vi "STM_Status.vi"() -> ()   [LabVIEW 2014]
uses:
  <userlib>/Nanonis Prog Interface V5/Nanonis Prog Interface.lvlib
panel:
  out "max value STM":dbl=1.6219152410013038e-10
  out "max value prep":dbl=2.1490820234504326e-10
  in  "Emission Current":u16(ring) items=["10", "1", "0.1"]
  out "STM [mBar]":dbl=1.554608664022794e-10 format="%#.2g"
  out "Prep [mBar]":dbl=2.1460036525589032e-10 format="%#.2g"
  out "Pressure":cluster{timestamp[], dbl[]}[](graph)=[{[timestamp(3559596166.680481 s since 1904-01-01), timestamp(3559596187.2546577 s since 1904-01-01)], [1.6219152410013038e-10, 1.5602781566759205e-10]}, {[timestamp(3559596166.680481 s since 1904-01-01), timestamp(3559596187.2546577 s since 1904-01-01)], [2.1490820234504326e-10, 2.1469723221478887e-10]}]
  in  "Resolution P":dbl=0.1
  in  "force update":dbl=20.0
  out "Cryo [K]":dbl=4.220807947684371 format="%#.2g"
  out "STM [K]":dbl=4.597361930995425 format="%#.2g"
  in  "Resolution Temp":dbl=0.1
  out "Temperature":cluster{timestamp[], dbl[]}[](graph)=[{[timestamp(3559596166.680481 s since 1904-01-01), timestamp(3559596187.2546577 s since 1904-01-01)], [4.221571920530717, 4.221402148787085]}, {[timestamp(3559596166.680481 s since 1904-01-01), timestamp(3559596187.2546577 s since 1904-01-01)], [4.572162263240161, 4.589400389803902]}]
  in  "Clear chart":bool
  in  "stop":bool
  in  "refresh":dbl=1.0
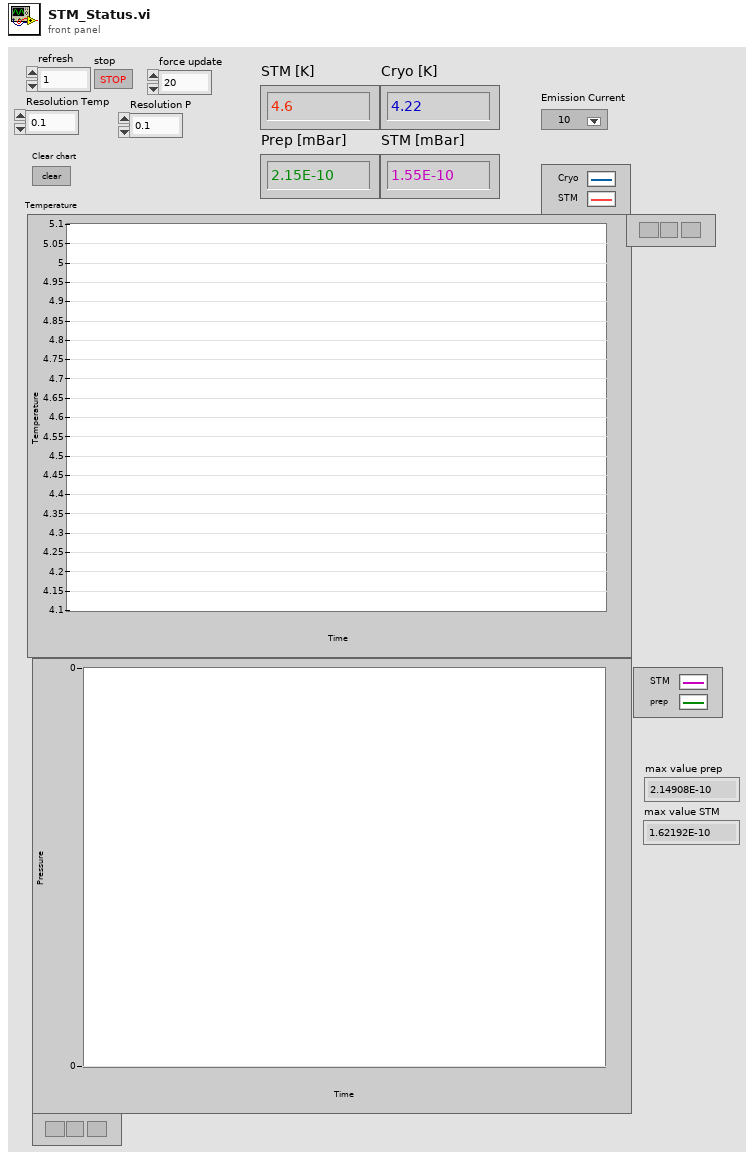
[diagram p1: front panel]
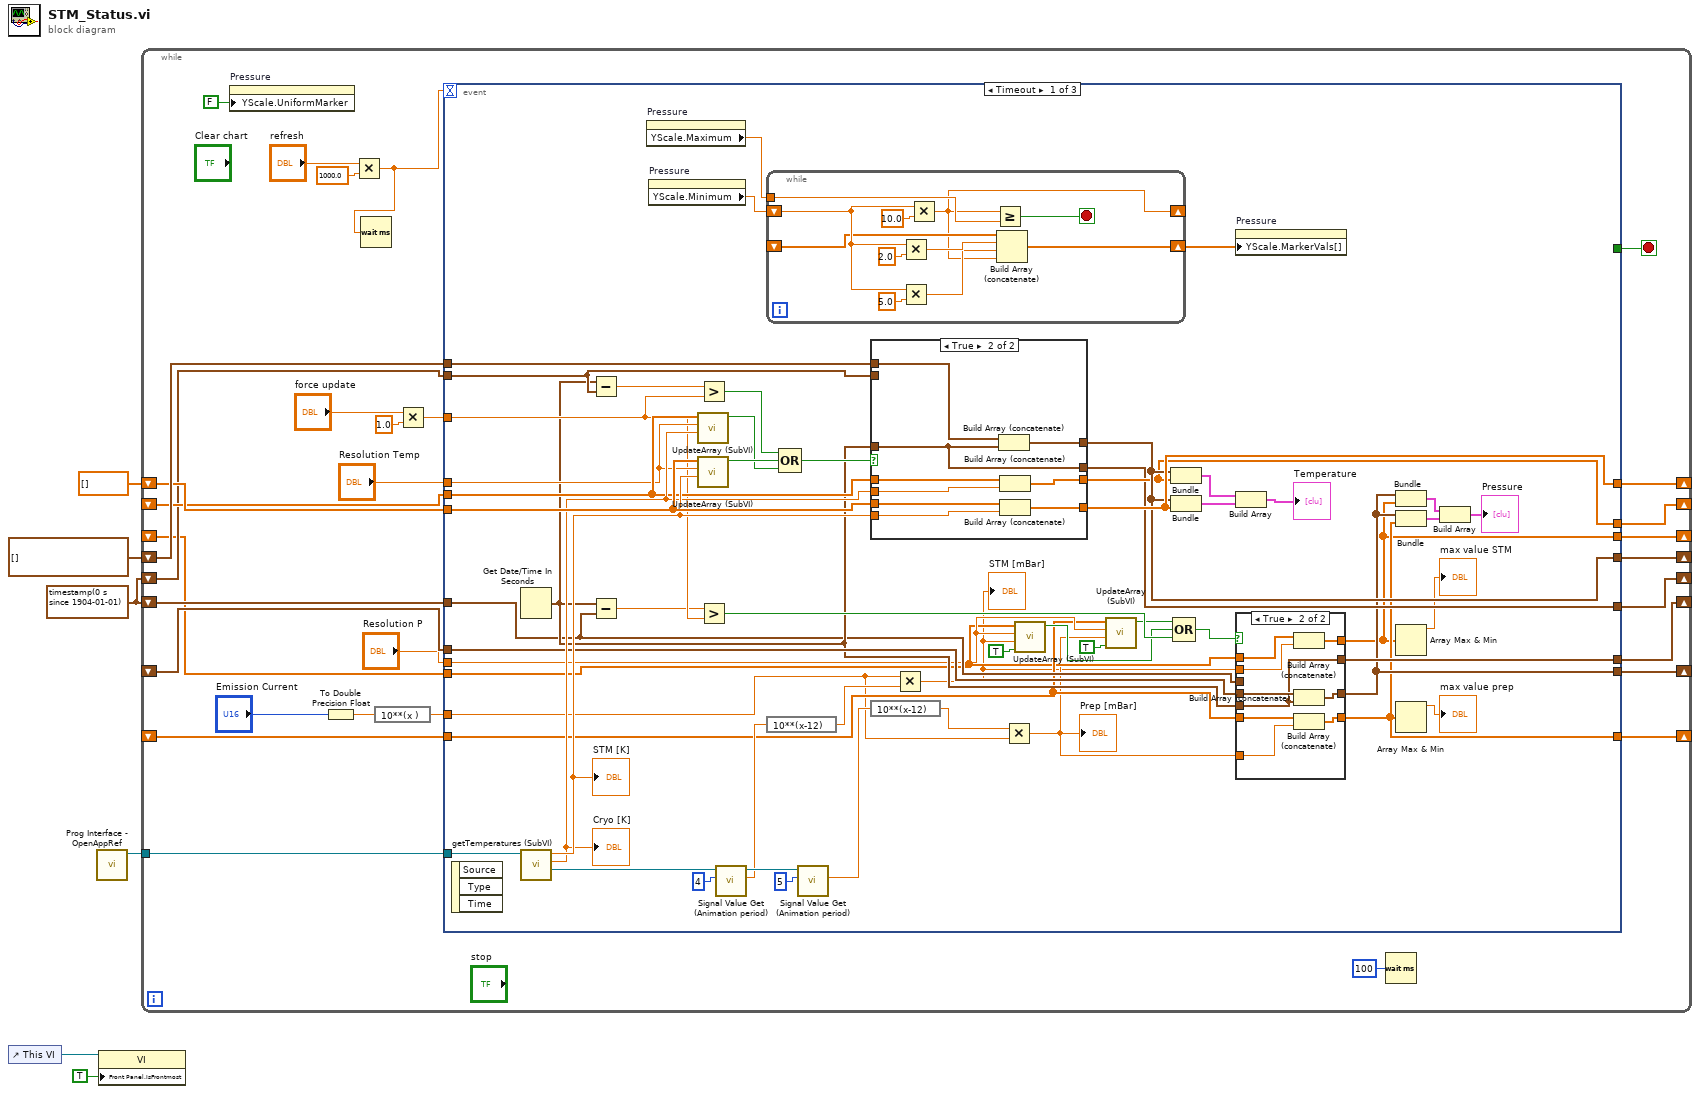
[diagram p0: block diagram]
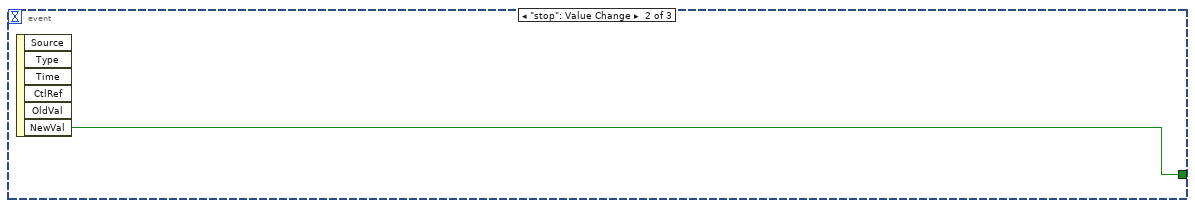
[diagram p4: hidden frame]
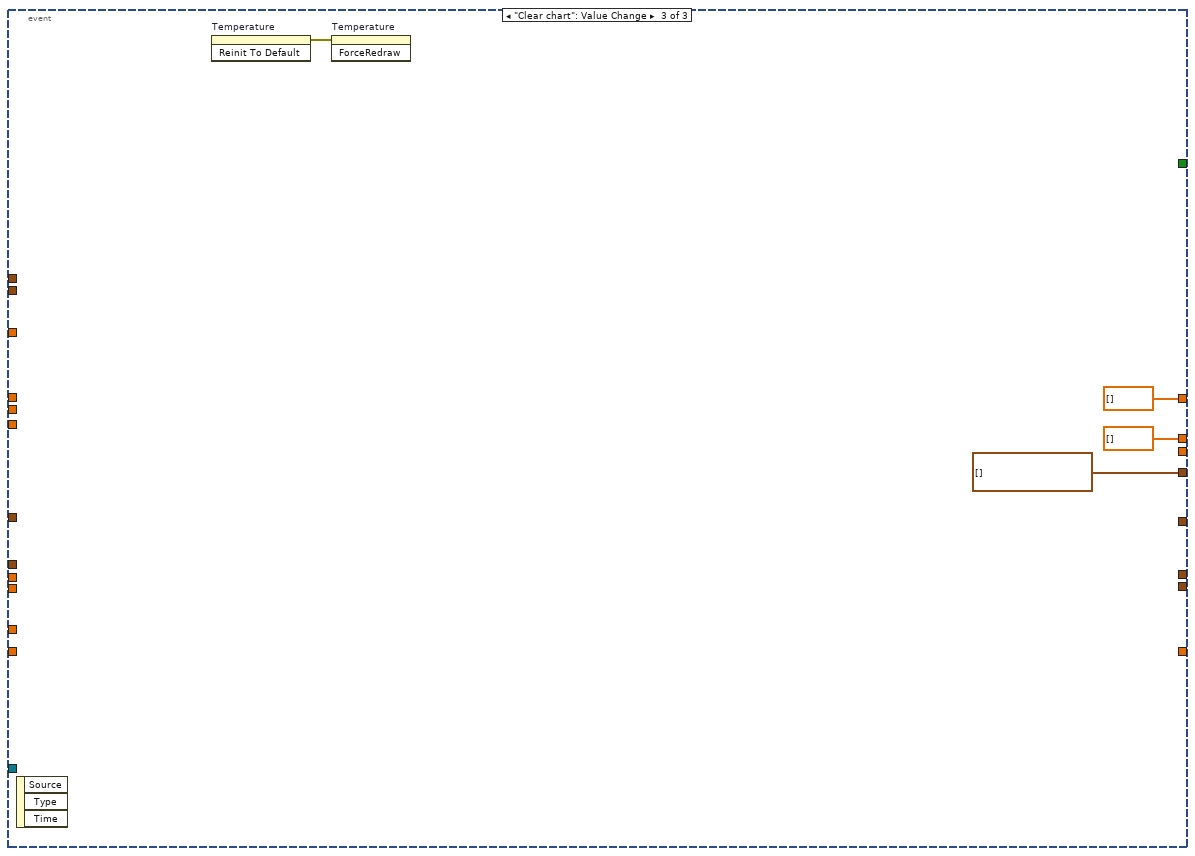
[diagram p5: hidden frame]
diagram:
  w3 = timestamp(0 s since 1904-01-01) ("seconds since 1Jan1904")
  n1 = control-ref of="This VI"() -> (w2:refnum<vi>)
  n2 = call <userlib>:"Prog Interface - OpenAppRef.vi"() -> ("Application reference"=w4:refnum<vi>)  [unwired: 6 in, 1 out]
  n3 = property class="VI"(reference=w2, "Front Panel.IsFrontmost"=TRUE ("Front Panel Window:Is Frontmost")) -> ()  [unwired: 1 in, 2 out]
  n4 = while {
    tunnel: w4 -> [w28]
    shift-right: [w35] -> _
    shift-left: timestamp[] [] -> [w31]
    shift-right: [w34] -> _
    shift-left: dbl[] [] -> [w30]
    shift-right: [w33] -> _
    shift-left: _ -> [w29]
    shift-right: [w26] -> _
    shift-left: w3 -> [w25]
    shift-right: [w21] -> _
    shift-left: _ -> [w20]
    shift-right: [w19] -> _
    shift-left: w3 -> [w18]
    shift-right: [w17] -> _
    shift-left: _ -> [w16]
    shift-right: [w15] -> _
    shift-left: _ -> [w14]
    stop <- w32 stop-if-true
    n5 = property on="Pressure" class="XYGraph (strict)"("YScale.UniformMarker"=FALSE ("Y Scale.Uniform Marker Spacing?")) -> ()  [unwired: 2 in, 2 out]
    n6 = To Double Precision Float(number="Emission Current") -> (double precision float=w9:dbl)
    n7 = Multiply(x="refresh", y=1000.0) -> (x*y=w8:dbl)
    n8 = Wait (ms)(milliseconds to wait=w8) -> ()  [unwired: 1 out]
    n9 = expression code="10**(x )"(w9) -> (w10:dbl)
    n10 = Multiply(x="force update", y=1.0) -> (x*y=w22:dbl)
    n11 = event shown="[0] Timeout" {
      selector: _ -> [_ _ _]
      dyn-events: _ -> [_ _ _]
      timeout: w8 -> [_ _ _]
      tunnel: [w88 _ timestamp[] []] -> w35
      tunnel: [w89 _ dbl[] []] -> w34
      tunnel: [w87 _ dbl[] []] -> w33
      tunnel: [_ w132 _] -> w32
      tunnel: w31 -> [w91 _ _]
      tunnel: w30 -> [w86 _ _]
      tunnel: w29 -> [w83 _ _]
      tunnel: w28 -> [w90 _ _]
      tunnel: "Resolution Temp" -> [w82 _ _]
      tunnel: [w77 _ _] -> w26
      tunnel: w25 -> [w75 _ _]
      tunnel: w22 -> [w69 _ _]
      tunnel: [w61 _ _] -> w21
      tunnel: w20 -> [w71 _ _]
      tunnel: [w67 _ _] -> w19
      tunnel: w18 -> [w66 _ _]
      tunnel: [w40 _ _] -> w17
      tunnel: w16 -> [w52 _ _]
      tunnel: [w42 _ _] -> w15
      tunnel: w14 -> [w53 _ _]
      tunnel: "Resolution P" -> [w54 _ _]
      tunnel: w10 -> [w45 _ _]
      event Timeout {
        n12 = event-data() -> ()  [unwired: 1 in, 3 out]
        n13 = Get Date/Time In Seconds() -> (seconds since 1Jan1904=w68:timestamp)
        n14 = call "getTemperatures (SubVI).vi"("Application in"=w90) -> ("Application ref out"=w58:refnum<vi>, "TCryo"=w84:dbl, "TSTM"=w85:dbl)  [unwired: 7 in, 1 out]
        "STM [K]" <- w85
        "Cryo [K]" <- w84
        n15 = Subtract(x=w68, y=w75) -> (x-y=w78:dbl)
        n16 = Subtract(x=w68, y=w66) -> (x-y=w65:dbl)
        n17 = property on="Pressure" class="XYGraph (strict)"() -> ("YScale.Maximum"=w38:dbl)  [unwired: 2 in, 2 out]
        n18 = property on="Pressure" class="XYGraph (strict)"() -> ("YScale.Minimum"=w44:dbl)  [unwired: 2 in, 2 out]
        n19 = call "UpdateArray (SubVI).vi"("Temp1"=w84, "Resolution"=w82, "Array"=w83) -> ("x > y?"=w79:bool)  [unwired: 8 in]
        n20 = call "UpdateArray (SubVI).vi"("Temp1"=w85, "Resolution"=w82, "Array"=w86) -> ("x > y?"=w80:bool)  [unwired: 8 in]
        n21 = Greater?(x=w78, y=w69) -> (0:w76:bool)
        n22 = Greater?(x=w65, y=w69) -> (0:w70:bool)
        n23 = call <userlib>:"Signal Value Get (Animation period).vi"("Signal index (0-47)"=i8 4, "Application ref in"=w58) -> ("Signal value"=w59:sgl, "Application ref out"=w74:refnum<vi>)  [unwired: 6 in, 1 out]
        n24 = while {
          tunnel: w38 -> [w104]
          shift-right: [w95] -> _
          shift-left: w44 -> [w100]
          shift-right: [w98] -> w43
          shift-left: _ -> [w99]
          stop <- w105 stop-if-true
          n25 = Multiply(x=w100, y=2.0) -> (x*y=w97:dbl)
          n26 = Multiply(x=w100, y=5.0) -> (x*y=w96:dbl)
          n27 = Multiply(x=w100, y=10.0) -> (x*y=w95:dbl)
          n28 = Greater Or Equal?(x=w95, y=w104) -> (x >= y?=w105:bool)
          n29 = Build Array (concatenate)(w99, w97, w96, w95) -> (w98:dbl[])
        }
        n30 = expression code="10**(x-12)"(w59) -> (w50:sgl)
        n31 = Compound Arithmetic op=OR(w76, w80, w79) -> (w81:bool)
        n32 = call <userlib>:"Signal Value Get (Animation period).vi"("Signal index (0-47)"=i8 5, "Application ref in"=w74) -> ("Signal value"=w57:sgl)  [unwired: 6 in, 2 out]
        n33 = case shown="True" w81 {
          tunnel: w68 -> [_ w123]
          tunnel: w91 -> [w122 w131]
          tunnel: [w120 w130] -> w89
          tunnel: [w122 w129] -> w88
          tunnel: [w121 w128] -> w87
          tunnel: w86 -> [w120 w127]
          tunnel: w85 -> [_ w126]
          tunnel: w84 -> [_ w125]
          tunnel: w83 -> [w121 w124]
          tunnel: [w119 w123] -> w77
          tunnel: w75 -> [w119 _]
          frame False {
          }
          frame True {
            n34 = Build Array (concatenate)(w131, w123) -> (w129:timestamp[])
            n35 = Build Array (concatenate)(w124, w125) -> (w128:dbl[])
            n36 = Build Array (concatenate)(w127, w126) -> (w130:dbl[])
          }
        }
        n37 = expression code="10**(x-12)"(w57) -> (w51:sgl)
        n38 = Multiply(x=w45, y=w50) -> (x*y=w46:dbl)
        "STM [mBar]" <- w46
        n39 = Multiply(x=w51, y=w45) -> (x*y=w47:dbl)
        "Prep [mBar]" <- w47
        n40 = call "UpdateArray (SubVI).vi"("log"=TRUE, "Temp1"=w46, "Resolution"=w54, "Array"=w52) -> ("x > y?"=w55:bool)  [unwired: 7 in]
        n41 = call "UpdateArray (SubVI).vi"("log"=TRUE, "Temp1"=w47, "Resolution"=w54, "Array"=w53) -> ("x > y?"=w56:bool)  [unwired: 7 in]
        n42 = Bundle(w88, w87) -> (w94:cluster{timestamp[], dbl[]})  [unwired: 1 in]
        n43 = Bundle(w88, w89) -> (w93:cluster{timestamp[], dbl[]})  [unwired: 1 in]
        n44 = Compound Arithmetic op=OR(w56, w55, w70) -> (w60:bool)
        n45 = property on="Pressure" class="XYGraph (strict)"("YScale.MarkerVals[]"=w43) -> ()  [unwired: 2 in, 2 out]
        n46 = Build Array(w94, w93) -> (→"Temperature":cluster{timestamp[], dbl[]}[])
        n47 = case shown="True" w60 {
          tunnel: w68 -> [_ w111]
          tunnel: w71 -> [w109 w118]
          tunnel: [w107 w117] -> w42
          tunnel: [w109 w116] -> w61
          tunnel: [w108 w115] -> w40
          tunnel: w53 -> [w107 w114]
          tunnel: w47 -> [_ w110]
          tunnel: w46 -> [_ w113]
          tunnel: w52 -> [w108 w112]
          tunnel: [w106 w111] -> w67
          tunnel: w66 -> [w106 _]
          frame False {
          }
          frame True {
            n48 = Build Array (concatenate)(w112, w113) -> (w115:dbl[])
            n49 = Build Array (concatenate)(w118, w111) -> (w116:timestamp[])
            n50 = Build Array (concatenate)(w114, w110) -> (w117:dbl[])
          }
        }
        n51 = Bundle(w61, w40) -> (w64:cluster{timestamp[], dbl[]})  [unwired: 1 in]
        n52 = Bundle(w61, w42) -> (w63:cluster{timestamp[], dbl[]})  [unwired: 1 in]
        n53 = Array Max & Min(array=w40) -> (max value=→"max value STM":dbl)  [unwired: 3 out]
        n54 = Array Max & Min(array=w42) -> (max value=→"max value prep":dbl)  [unwired: 3 out]
        n55 = Build Array(w64, w63) -> (→"Pressure":cluster{timestamp[], dbl[]}[])
      }
      event "stop": Value Change {
        n56 = event-data() -> ("NewVal"=w132:bool)  [unwired: 1 in, 5 out]
      }
      event "Clear chart": Value Change {
        n57 = event-data() -> ()  [unwired: 1 in, 3 out]
        n58 = invoke on="Temperature" class="XYGraph (strict)" method="Reinit To Default"() -> (error out=w133:errorcluster)  [unwired: 3 in, 2 out]
        n59 = invoke on="Temperature" class="XYGraph (strict)" method="ForceRedraw"(error in=w133) -> ()  [unwired: 2 in, 3 out]
      }
    }
    n60 = Wait (ms)(milliseconds to wait=u32 100) -> ()  [unwired: 1 out]
  }
